vi "Host - Launch TCP Serial VIs (SubVI).vi"() -> (1 "TCP Serial Data":string[][](array[string]), 2 "TCP Serial Ref":refnum<vi>[](array[refnum]))   [LabVIEW 2021]
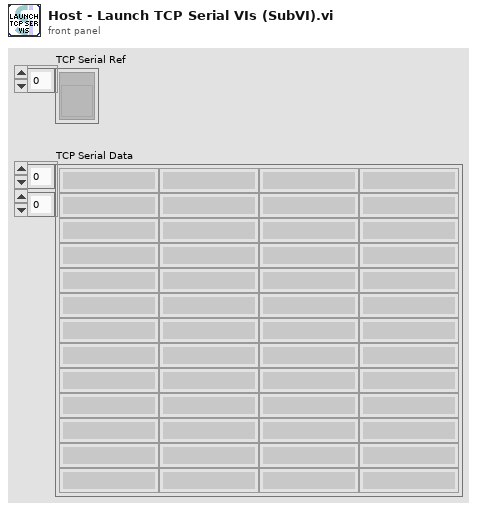
[diagram p1: front panel]
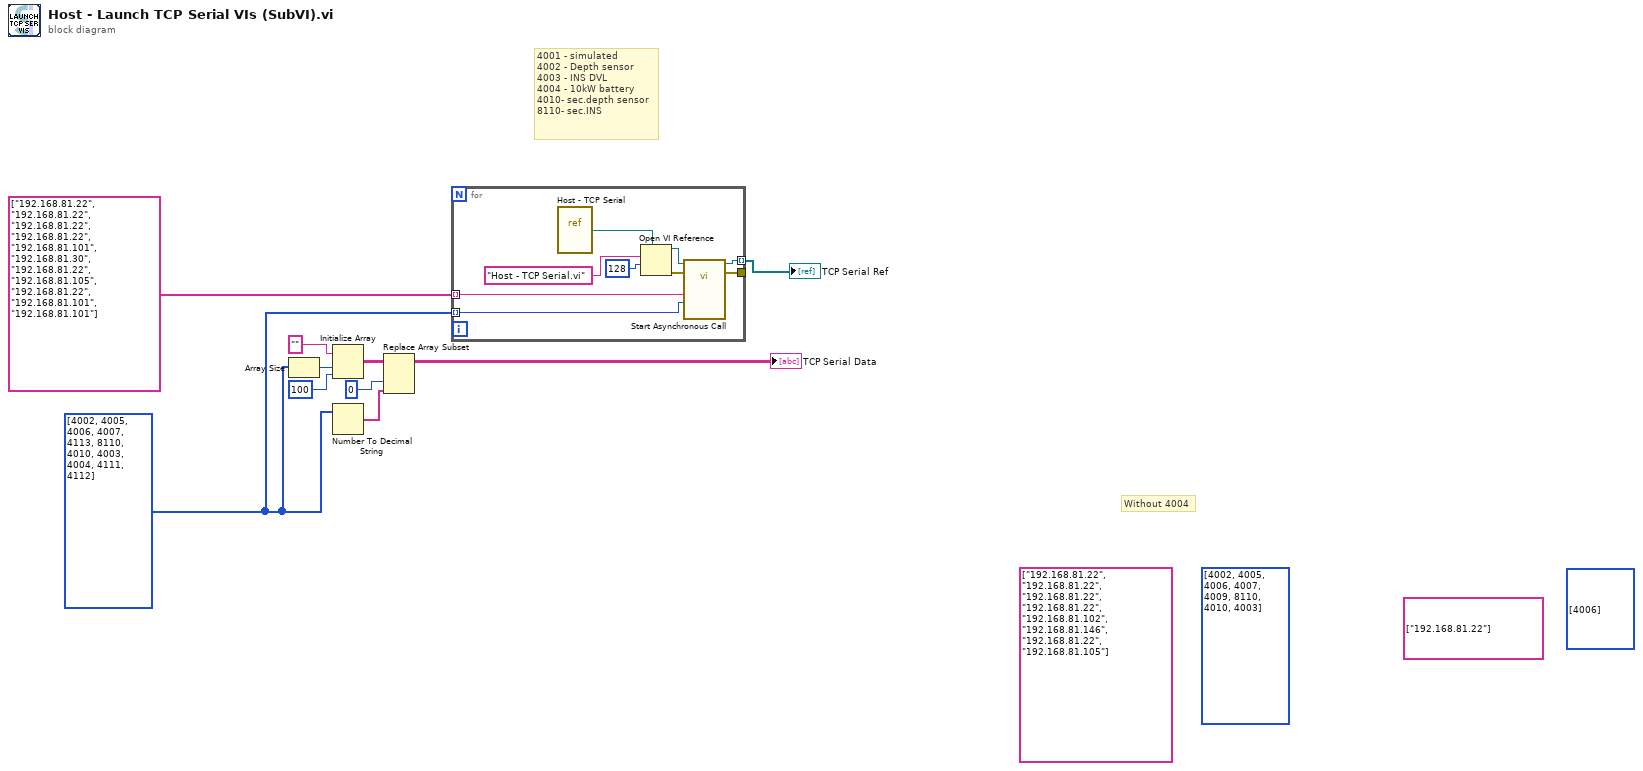
[diagram p0: block diagram]
diagram:
  w1 = u16[] [4002, 4005, 4006, 4007, 4113, 8110, 4010, 4003, 4004, 4111, 4112] ("Addresses")
  (unwired) string[] ["192.168.81.22"] ("Addresses")
  (unwired) u16[] [4006] ("Addresses")
  (unwired) string[] ["192.168.81.22", "192.168.81.22", "192.168.81.22", "192.168.81.22", "192.168.81.102", "192.168.81.146", "192.168.81.22", "192.168.81.105"] ("Addresses")
  (unwired) u16[] [4002, 4005, 4006, 4007, 4009, 8110, 4010, 4003] ("Addresses")
  # "Without 4004"
  # "4001 - simulated\n4002 - Depth sensor\n4003 - INS DVL\n4004 - 10kW battery\n4010- sec.depth sensor\n8110- sec.INS"
  n1 = Array Size(array=w1) -> (size(s)=w5:i32)
  n2 = Initialize Array("" ("PageLabel"), w5, 100 ("dimension size")) -> (w7:string[][])
  n3 = Number To Decimal String(number=w1) -> (decimal integer string=w8:string[])  [unwired: 1 in]
  n4 = Replace Array Subset(array=w7, new element=w8, index (col)=0 ("disabled index (col)")) -> (→"TCP Serial Data":string[][])  [unwired: 1 in]
  n5 = for {
    tunnel: [w15] -> w3 mode=indexing
    tunnel: [w14] -> _
    tunnel: string[] ["192.168.81.22", "192.168.81.22", "192.168.81.22", "192.168.81.22", "192.168.81.101", "192.168.81.30", "192.168.81.22", "192.168.81.105", "192.168.81.22", "192.168.81.101", "192.168.81.101"] ("Addresses") -> [w12] mode=indexing
    tunnel: w1 -> [w11] mode=indexing
    n6 = vi-ref "Host - TCP Serial.vi"() -> (w18:refnum<vi>)
    n7 = Open VI Reference(type specifier VI Refnum (for type only)=w18, vi path="Host - TCP Serial.vi", options=128) -> (vi reference=w19:refnum<vi>, error out=w13:errorcluster)  [unwired: 3 in]
    n8 = call-by-ref "Start Asynchronous Call"(reference=w19, error in=w13, "port"=w11, "address"=w12) -> (reference out=w15:refnum<vi>, error out=w14:errorcluster)  [unwired: 10 in]
  }
  "TCP Serial Ref" <- w3
